vi "HEWH Reset MW100.vi"(8 "error in (no error)":errorcluster, 11 "MW100 VISA In":refnum<visa-resource-name>) -> (0 "error out":errorcluster, 3 "MW100 VISA Out":refnum<visa-resource-name>)   [LabVIEW 2016]
panel:
  out "Retries":i32
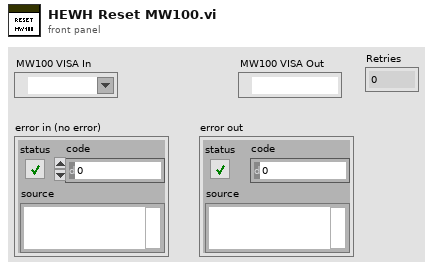
[diagram p1: front panel]
types:
  T1 = enum16{"Computation Start", "Computation stop", "Reset Computation", "Clear Computation"}[]
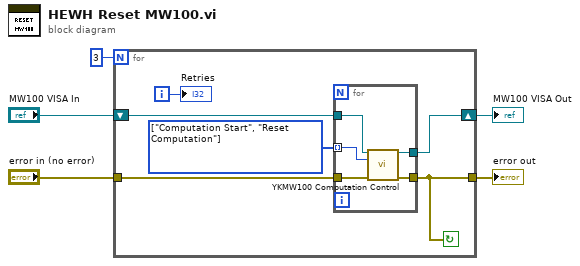
[diagram p0: block diagram]
diagram:
  n1 = for {
    N: 3 -> [_]
    shift-right: [w9] -> w4
    shift-left: "MW100 VISA In" -> [w11]
    tunnel: "error in (no error)" -> [w7]
    tunnel: [w6] -> w1
    i -> [w8]
    stop <- w6 continue-if-true
    w10 = T1 [enum."Computation Start", enum."Reset Computation"] items=["Computation Start", "Computation stop", "Reset Computation", "Clear Computation"]
    n2 = for {
      tunnel: w11 -> [w16]
      tunnel: w10 -> [w15] mode=indexing
      tunnel: [w14] -> w9
      tunnel: [w13] -> w6
      tunnel: w7 -> [w12]
      n3 = call "YKMW100 Computation Control.vi"("VISA session"=w16, "Mode"=w15, "error in (no error)"=w12) -> ("dup VISA session"=w14:refnum<visa-resource-name>, "error out"=w13:errorcluster)  [unwired: 11 in]
    }
    "Retries" <- w8
  }
  "error out" <- w1
  "MW100 VISA Out" <- w4
